vi "事件结构.vi"() -> ()   [LabVIEW 2018]
panel:
  in  "停止":bool
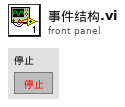
[diagram p1: front panel]
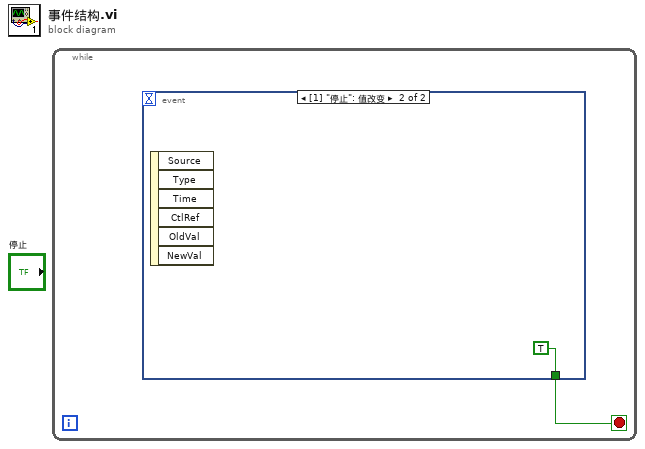
[diagram p0: block diagram]
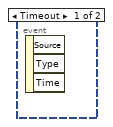
[diagram p2: hidden frame]
diagram:
  n1 = while {
    stop <- w1 stop-if-true
    n2 = event shown="[1] \"停止\": 值改变" {
      selector: _ -> [_ _]
      dyn-events: _ -> [_ _]
      timeout: _ -> [_ _]
      tunnel: [_ TRUE] -> w1
      event Timeout {
        n3 = event-data() -> ()  [unwired: 1 in, 3 out]
      }
      event "停止": Value Change {
        n4 = event-data() -> ()  [unwired: 1 in, 6 out]
      }
    }
  }
